vi "Read Display Name.vi"(8 "error in (no error)":errorcluster, 11 "External Calibration Operator in":refnum<class "External Calibration Operator.lvclass">) -> (0 "error out":errorcluster, 2 "display name":string, 3 "External Calibration Operator out":refnum<class "External Calibration Operator.lvclass">)   [LabVIEW 2019, in "External Calibration Operator.lvclass"]
uses:
  External Calibration Operator.lvclass
  External Calibration Operator.lvclass/External Calibration Operator.ctl
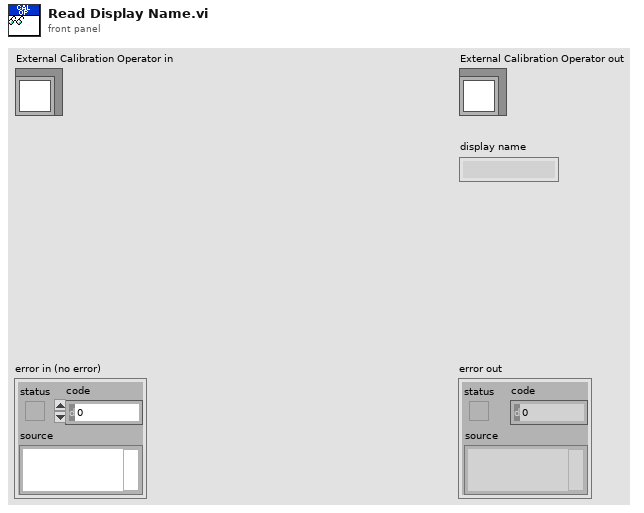
[diagram p1: front panel]
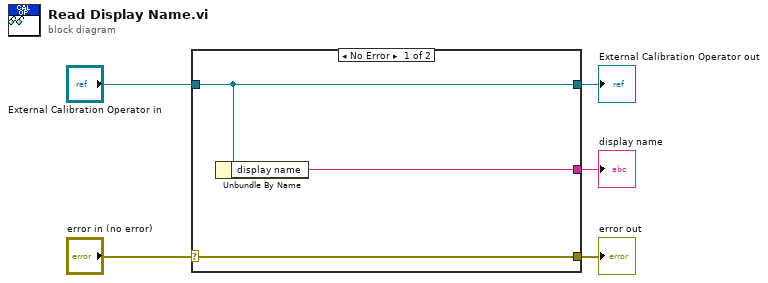
[diagram p0: block diagram]
diagram:
  n1 = case shown="No Error" "error in (no error)" {
    selector: "error in (no error)" -> [w8 w9]
    tunnel: [w8 w9] -> w4
    tunnel: [w7 w10] -> w2
    tunnel: "External Calibration Operator in" -> [w7 w10]
    tunnel: [w6 _] -> w1
    frame No Error {
      n2 = Unbundle By Name(w7) -> ("display name"=w6:string)
    }
    frame Error {
    }
  }
  "error out" <- w4
  "External Calibration Operator out" <- w2
  "display name" <- w1
